vi "Write to File.vi"(7 "Section Name":string, 8 "error in (no error)":errorcluster, 10 "INI Ref":T1, 11 "Keyboard Action in":refnum<class "Keyboard Action.lvclass">) -> (0 "error out":errorcluster, 2 "INI Ref out":T1, 3 "Keyboard Action out":refnum<class "Keyboard Action.lvclass">)   [LabVIEW 2020, in "MacroAssert.lvlib" / "Keyboard Action.lvclass"]
doc: "Writes associated parameters to the file identified by <B>INI Ref</B>."
uses:
  Keyboard Action.lvclass
  <vilib>/Utility/config.llb/Config Data RefNum.ctl
  <vilib>/Utility/error.llb/Error Cluster From Error Code.vi
  <vilib>/Utility/config.llb/Write Key (String).vi
  <vilib>/Utility/config.llb/Write Key (U32).vi
  <vilib>/Utility/config.llb/Write Key (I32).vi
  <vilib>/Utility/config.llb/Write Key (Boolean).vi
  Action Step/Action Step.lvclass
  SubVIs/Custom Errors/Custom Errors.lvlib
  <vilib>/Utility/config.llb/NI_LVConfig.lvlib
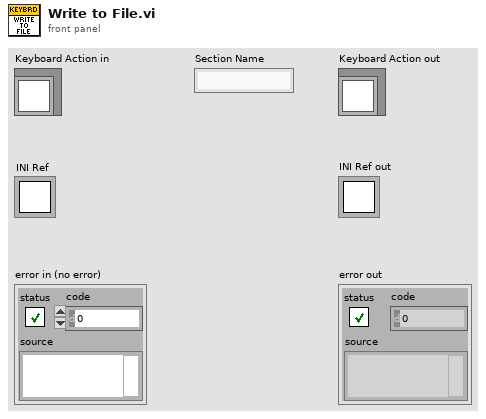
[diagram p1: front panel]
types:
  T1 = typedef "NI_LVConfig.lvlib/Config Data RefNum.ctl" = refnum<k1>
  T2 = typedef "MacroAssert.lvlib/Keyboard Action.lvclass/Keyboard Action Type.ctl" = enum16{"Key Press", "Key Down", "Key Up"}
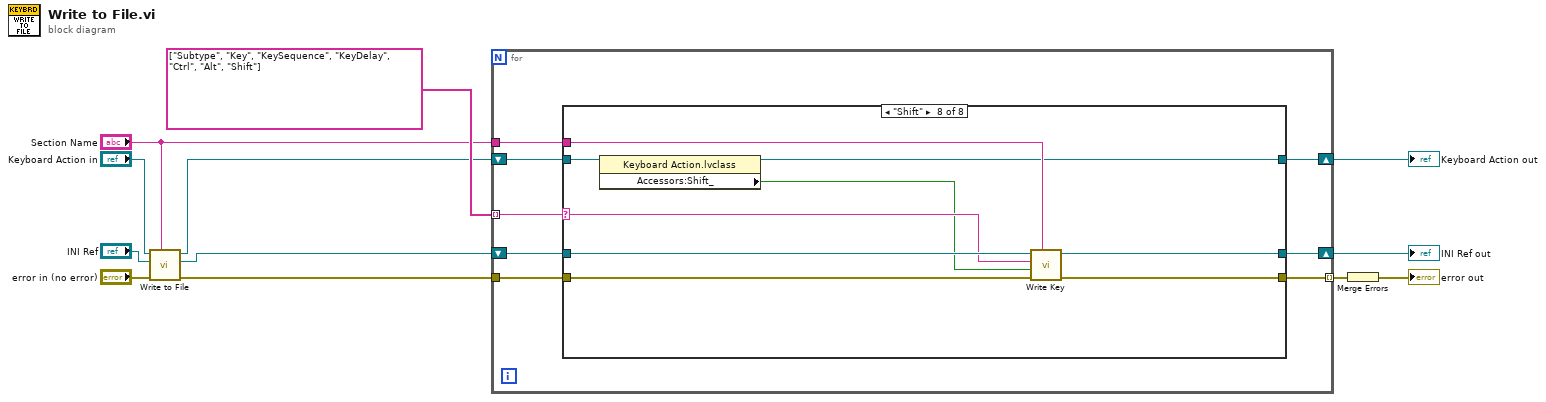
[diagram p0: block diagram]
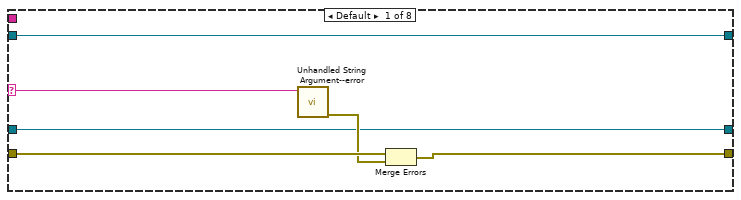
[diagram p2: hidden frame]
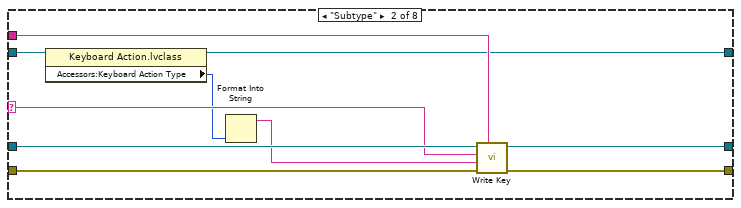
[diagram p3: hidden frame]
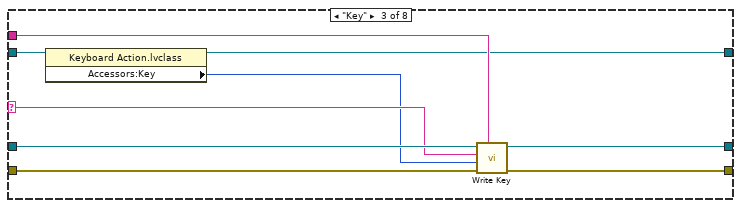
[diagram p4: hidden frame]
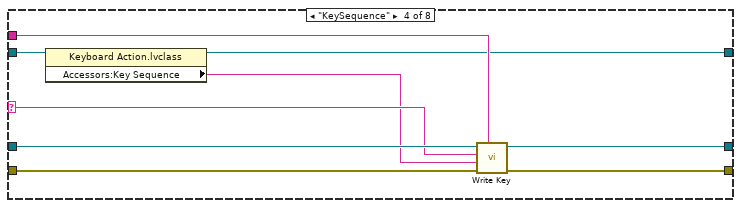
[diagram p5: hidden frame]
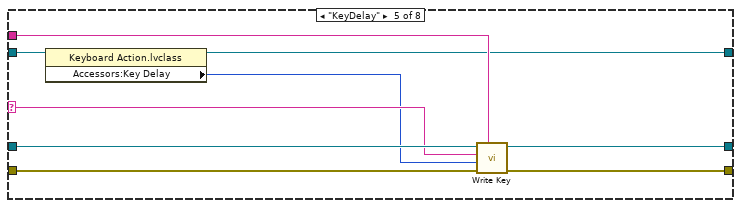
[diagram p6: hidden frame]
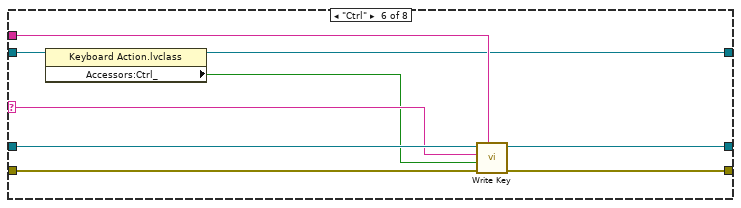
[diagram p7: hidden frame]
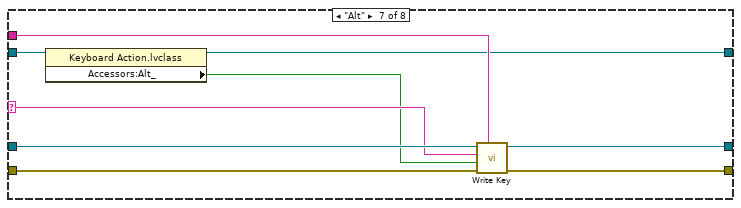
[diagram p8: hidden frame]
diagram:
  n1 = call-parent "Write to File.vi"("Section Name"="Section Name", "error in (no error)"="error in (no error)", "INI Ref"="INI Ref", "Step in"="Keyboard Action in") -> ("error out"=w11:errorcluster, "INI Ref out"=w7:T1, "Step out"=w3:refnum<class "Keyboard Action.lvclass">)  [unwired: 5 in]
  n2 = for {
    tunnel: string[] ["Subtype", "Key", "KeySequence", "KeyDelay", "Ctrl", "Alt", "Shift"] -> [w16] mode=indexing
    tunnel: w11 -> [w20]
    tunnel: "Section Name" -> [w15]
    shift-right: [w13] -> w2
    shift-left: w3 -> [w14]
    tunnel: [w19] -> w4 mode=indexing
    shift-right: [w17] -> w8
    shift-left: w7 -> [w18]
    n3 = case shown="\"Shift\"" w16 {
      selector: w16 -> [w21 w31 w40 w49 w58 w67 w76 w85]
      tunnel: w20 -> [w26 w36 w45 w54 w63 w72 w81 w90]
      tunnel: w15 -> [_ w32 w41 w50 w59 w68 w77 w86]
      tunnel: w14 -> [w22 w30 w39 w48 w57 w66 w75 w84]
      tunnel: [w22 w27 w38 w47 w56 w65 w74 w83] -> w13
      tunnel: [w24 w35 w44 w53 w62 w71 w80 w89] -> w19
      tunnel: w18 -> [w23 w34 w43 w52 w61 w70 w79 w88]
      tunnel: [w23 w33 w42 w51 w60 w69 w78 w87] -> w17
      frame Default {
        n4 = call "Unhandled String Argument--error.vi"("Argument"=w21) -> ("error out"=w25:errorcluster)  [unwired: 10 in]
        n5 = Merge Errors(w26, w25) -> (w24:errorcluster)
      }
      frame "Subtype" {
        n6 = property class="Keyboard Action.lvclass"(reference=w30) -> (reference out=w27:refnum<class "Keyboard Action.lvclass">, "Accessors:Keyboard Action Type"=w29:T2)  [unwired: 1 in, 1 out]
        n7 = Format Into String(w29) -> (resulting string=w28:string)  [unwired: 3 in, 1 out]
        n8 = call-poly <vilib>:"Write Key.vi"("section"=w32, "error in (no error)"=w36, "value"=w28, "key"=w31, "refnum"=w34) -> ("error out"=w35:errorcluster, "refnum out"=w33:T1)  [unwired: 4 in, 1 out]
      }
      frame "Key" {
        n9 = property class="Keyboard Action.lvclass"(reference=w39) -> (reference out=w38:refnum<class "Keyboard Action.lvclass">, "Accessors:Key"=w37:u8)  [unwired: 1 in, 1 out]
        n10 = call-poly <vilib>:"Write Key.vi"("section"=w41, "error in (no error)"=w45, "value"=w37, "key"=w40, "refnum"=w43) -> ("error out"=w44:errorcluster, "refnum out"=w42:T1)  [unwired: 4 in, 1 out]
      }
      frame "KeySequence" {
        n11 = property class="Keyboard Action.lvclass"(reference=w48) -> (reference out=w47:refnum<class "Keyboard Action.lvclass">, "Accessors:Key Sequence"=w46:string)  [unwired: 1 in, 1 out]
        n12 = call-poly <vilib>:"Write Key.vi"("section"=w50, "error in (no error)"=w54, "value"=w46, "key"=w49, "refnum"=w52) -> ("error out"=w53:errorcluster, "refnum out"=w51:T1)  [unwired: 4 in, 1 out]
      }
      frame "KeyDelay" {
        n13 = property class="Keyboard Action.lvclass"(reference=w57) -> (reference out=w56:refnum<class "Keyboard Action.lvclass">, "Accessors:Key Delay"=w55:i32)  [unwired: 1 in, 1 out]
        n14 = call-poly <vilib>:"Write Key.vi"("section"=w59, "error in (no error)"=w63, "value"=w55, "key"=w58, "refnum"=w61) -> ("error out"=w62:errorcluster, "refnum out"=w60:T1)  [unwired: 4 in, 1 out]
      }
      frame "Ctrl" {
        n15 = property class="Keyboard Action.lvclass"(reference=w66) -> (reference out=w65:refnum<class "Keyboard Action.lvclass">, "Accessors:Ctrl_"=w64:bool)  [unwired: 1 in, 1 out]
        n16 = call-poly <vilib>:"Write Key.vi"("section"=w68, "error in (no error)"=w72, "value"=w64, "key"=w67, "refnum"=w70) -> ("error out"=w71:errorcluster, "refnum out"=w69:T1)  [unwired: 4 in, 1 out]
      }
      frame "Alt" {
        n17 = property class="Keyboard Action.lvclass"(reference=w75) -> (reference out=w74:refnum<class "Keyboard Action.lvclass">, "Accessors:Alt_"=w73:bool)  [unwired: 1 in, 1 out]
        n18 = call-poly <vilib>:"Write Key.vi"("section"=w77, "error in (no error)"=w81, "value"=w73, "key"=w76, "refnum"=w79) -> ("error out"=w80:errorcluster, "refnum out"=w78:T1)  [unwired: 4 in, 1 out]
      }
      frame "Shift" {
        n19 = property class="Keyboard Action.lvclass"(reference=w84) -> (reference out=w83:refnum<class "Keyboard Action.lvclass">, "Accessors:Shift_"=w82:bool)  [unwired: 1 in, 1 out]
        n20 = call-poly <vilib>:"Write Key.vi"("section"=w86, "error in (no error)"=w90, "value"=w82, "key"=w85, "refnum"=w88) -> ("error out"=w89:errorcluster, "refnum out"=w87:T1)  [unwired: 4 in, 1 out]
      }
    }
  }
  "Keyboard Action out" <- w2
  "INI Ref out" <- w8
  n21 = Merge Errors(w4) -> (→"error out":errorcluster)
